vi "Big_LED_control.vi"() -> ()   [LabVIEW 2018]
uses:
  <instrlib>/niDCPower/nidcpower.llb/niDCPower Source Mode.ctl
  <instrlib>/niDCPower/nidcpower.llb/niDCPower Output Function.ctl
  D:/#msp/LV/LED_CONTROL_big_LED_ophir_20.12/AT lib/AmateurStepperMotor.dll
  AT lib/AmateurStepperMotor.dll
  <instrlib>/niDMM/nidmm.llb/niDMM Function.ctl
  <instrlib>/niDMM/nidmm.llb/niDMM Resolution in Digits.ctl
  <vilib>/Instr/_visa.llb/VISA Configure Serial Port (Instr).vi
  <instrlib>/niDMM/nidmm.llb/niDMM Configure Measurement Digits.vi
panel:
  in  "Tab Control 2":enum32{"Шаговик и офир", "Служебная область"}(tab)
  in  "milliseconds to wait":u32=1000
  in  "Go To":dbl
  out "Ophir 1 Char":dbl(graph)=7.0
  in  "DecelerationTime, s":dbl
  in  "AccelerationTime, s":dbl
  in  "HoldOn":bool
  in  "Ophir 1 units":string(combo)="1000" caption="Units"
  out "Ophir 1 Over Range":bool caption="Over Range"
  out "Ophir 1 Optical Power":dbl=7.0 caption="Power" format="%#_4g"
  out "Ophir 1 MAX":dbl=7.0200000000000005 caption="MAX" format="%#_5g"
  in  "Ophir 1 Clear":bool caption="Clear"
  in  "StepMultiplicationFactor":dbl=1.0
  in  "StepDivisor":i32(ring)=8 items=["D1"=1, "D2"=2, "D4"=4, "D8"=8, "D16"=16, "D32"=32]
  in  "Speed":dbl=1000.0
  in  "Погнали!":bool
  in  "Стоп GoTo":bool
  out "Готово":bool
  out "Position":dbl
  in  "Ophir 1 Info":u16(ring)=1 caption="Info" items=["Device : JUNO; s/n:903793", "Head : PD300R-3W   ; s/n:779628"]
  in  "new pos":dbl
  in  "set pos":bool
  out "Device Response":string="*\n"
  in  "Ophir 1 usb channel":i16 caption="usb channel"
  out "Ophir 1 dup Visa Session":refnum<visa-resource-name>="USB0::0x0BD3::0x0777::NI-VISA-60004::RAW" caption="dup Visa Session"
  in  "Ophir 1 Baud Rate (3:9600)":i16(ring)=3 caption="Baud Rate (3:9600)" items=["300", "1200", "4800", "9600", "19200", "38400"]
  out "Ophir 1 Real Optical Power":dbl=0.007 format="%.6e"
  in  "Ophir 1 GPIB Address (10)":string="10" caption="GPIB Address (10)"
  in  "Ophir 1 Port Number (default 2)":i16=1 caption="Port Number (default 2)" min=0 max=20
  in  "Ophir 1 Select Communication Protocol":u16(ring) caption="Select Communication Protocol" items=["USB", "RS232", "GPIB"]
  out "Ophir 1 error out":errorcluster caption="error out"
  in  "Ophir 1 error in (no error)":errorcluster caption="error in (no error)"
  in  "Ophir 1 Wait":u32=100 caption="Wait"
  out "IsOpen":bool=TRUE
  out "Ophir 1 Initialization":bool=TRUE caption="Initialization"
  in  "Tab Control":T1(tab)
  in  "POWER":bool
  in  "Стоп":bool
  in  "Resource Name":refnum<k15>="PXI1Slot2" caption="Источник питания"
  in  "Амперметр":refnum<k15>="PXI1Slot4" caption="NI DMM 1"
  in  "V_MB, V":dbl=5.0 caption="voltage level" format="%_6p"
  in  "curlim_V_MB, A":dbl=0.3 caption="current limit" format="%_6p"
  out "curmes_V_MB, A":dbl caption="measurement" format="%_6g"
  out "chart_0":dbl(graph)=-0.001986406197333734 caption="Waveform Chart 5"
  in  "voltlim_I_LED, V":dbl=2.0 caption="current limit" min=0.01 format="%_6p"
  in  "I_LED, A":dbl=0.005 caption="voltage level" format="%_6p"
  out "chart_1":dbl(graph) caption="Waveform Chart 5"
  out "voltmes_I_LED, V":dbl caption="measurement" format="%_6g"
  out "Current Char":dbl(graph)=0.0019995495676994324
  in  "Arduino":refnum<visa-resource-name>="COM14"
  in  "Сегменты":bool[](array[boolean])=[FALSE, FALSE, FALSE, FALSE, FALSE, FALSE, FALSE, FALSE, FALSE, FALSE, FALSE, FALSE, FALSE, FALSE, FALSE, FALSE, FALSE, FALSE]
  in  "Вольтметр":refnum<k15>="PXI1Slot5" caption="NI DMM 1"
  out "Voltage Char":dbl(graph)=nan
  in  "Port Name":string="COM7" caption="Порт шаговика"
  in  "wave_lenght":string="600"
  in  "Промер":bool caption="Промер сегмента"
  in  "NI DMM 1 Voltage Range 4":string(combo)="-1" caption="Range"
  in  "NI DMM 1 units 4":string(combo)="1" caption="Units"
  out "Voltage":dbl=nan format="%_6g"
  in  "NI DMM 1 Current Range 3":string(combo)="1" caption="Range"
  in  "NI DMM 1 units 3":string(combo)="1000" caption="Units"
  out "Current":dbl=0.0019995495676994324 format="%_6g"
  out "curmes_I_LED, A":dbl caption="measurement" format="%_6g"
  out "voltmes_V_MB, V":dbl caption="measurement" format="%_6g"
  out "Разряд":dbl
  out "+/-":bool
  out "Power off":bool=TRUE
  in  "Command":string="Anode"
  in  "Записать":bool
  out "measure output file refnum":refnum<file>
  out "Voltage, V":dbl=nan caption="Measurement" format="%.5f"
  out "Current, A":dbl=1.9995495676994324e-06 caption="Measurement" format="%.5f"
  out "Тип индикатора":string="Anode"
  out "chart_2":dbl(graph)=4.286668577189643e-07
  in  "V_RES, V":dbl caption="voltage level" format="%_6p"
  out "curmes_V_RES, A":dbl caption="measurement" format="%_6g"
  in  "curlim_V_RES, A":dbl=0.1 caption="current limit" min=0.01 format="%_6p"
  in  "measure path":path=path "D:/NI LabVIEW/MultiOpto/MultiOpto_1.2/Logs/SEL"
  out "Enum":enum16{"Exit", "4", "Промер", "2", "1"}(ring)
  out "№ об-ца":dbl=-1.0
  out "Темп-ра":dbl=-1.0
  out "Сегмент":string
  out "voltmes_V_RES, V":dbl caption="measurement" format="%_6g"
  in  "current level range":dbl format="%#.6p"
  # "Шаговик"
  # "Офир"
  # "Шаговик"
  # "Офир"
  # "position - это значение абсолютное"
  # "j"
  # "c"
  # "d"
  # "e"
  # "g"
  # "h"
  # "a"
  # "b"
  # "f"
  # "k"
  # "L"
  # "m"
  # "n"
  # "p"
  # "dp"
  # "all"
  # "V_MB 5 В\nогрничение 300 м\n\nV_LED 2,1 В\nограничение 200 м"
  # "единицы мА\nrange 1 А"
  # "1. каждый сегмент включаем по отдельности, резистором постраиваем ток до 10 мА\n2. напряжение V_LED при этом не меняется\n3. в такоом положении промеряем сегменты по отдельности\n4. для промера всего индикатора сразу подстраиваем напряжение при неизменном положении резисторов\n5. ток всех индикаторов = ток одного сегмента (10 мА) * число сегментов (15)\n6. добиваемся этого увеличением V_LED"
  # "единицы В\nrange AUTO"
  # "регклировка суммарного тока через индикатор"
  # "24.063\n\n     I          U\n20 мА  1.3 В\n20 мА  1.4 В\n 7 мА   1.15 В"
  # "24.064\n\n     I          U\n10 мА  2 В\n10 мА  2.15 В\n 7 мА   1.9 В"
  # "автоматизировать подбор напряжения по известному максимальному напряжению и току. ОС по току сегмента"
  # "Р1:  +25°C\nР2:  - 60°C\nР3:  +85°C"
  # "регулировать ток в зависимости от температуры.\nс ростом температуры растет ток.\nпид-регулятор??"
  # "0. ввести номер образца\n1. включить нужный сегмент\n2. ввести его в поле справа\n3. вести температуру в поле слева\n4. нажать кнопку \"промер сегмента\""
  # "\"опрашивать кнопки не чаще, чем раз в секунду. сейчас кликать можно чаще, они загорятся, но ничего не произойдет\""
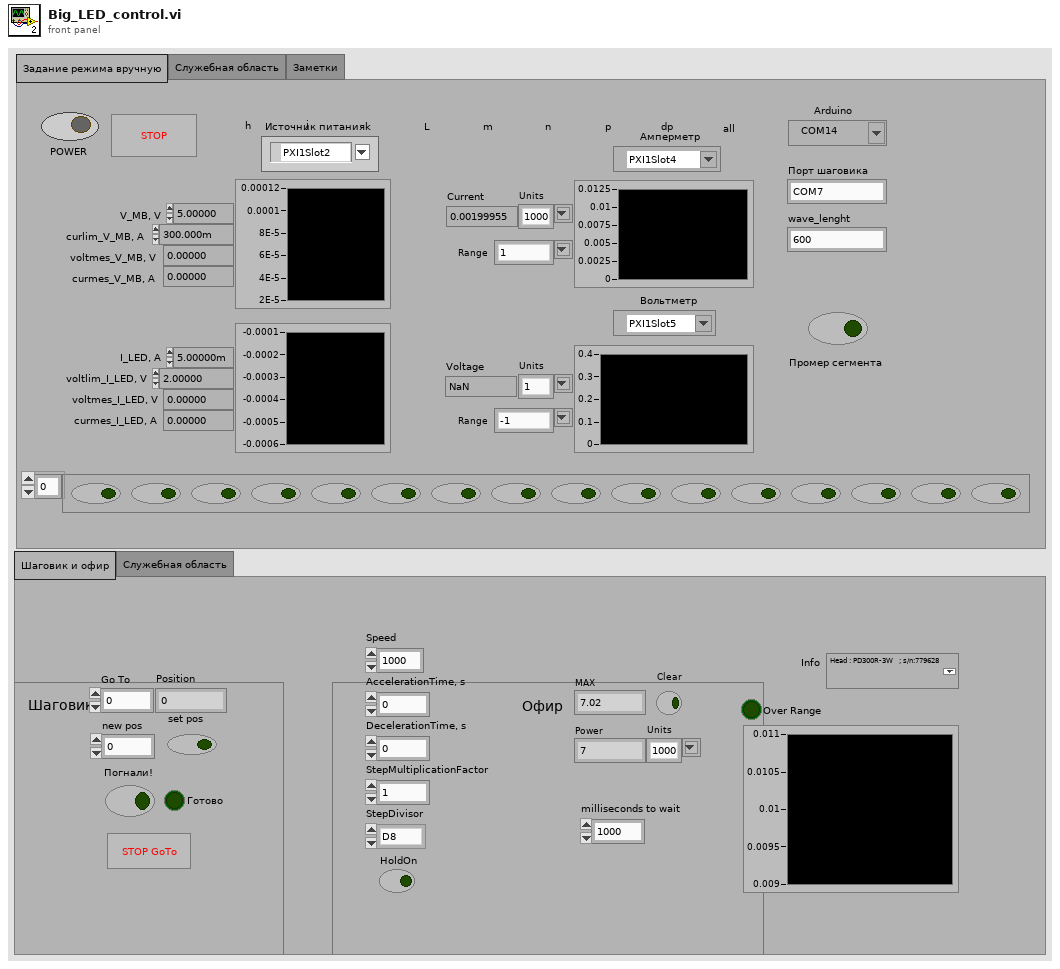
[diagram p1: front panel]
types:
  T1 = enum32{"Задание режима вручную", "Служебная область", "Заметки"}
  T2 = enum16{"open", "replace", "create", "open or create", "replace or create", "replace or create with confirmation"}
  T3 = typedef "niDCPower Output Function.ctl" = i32
  T4 = typedef "niDCPower Source Mode.ctl" = i32
  T5 = typedef "niDMM Function.ctl" = enum16{"DC Volts", "AC Volts", "DC Current", "AC Current", "2-wire Resistance", "4-wire Resistance", "Diode", "Frequency", "Period", "AC Volts DC Coupled", "Capacitance", "Inductance", "Temperature"}
  T6 = typedef "niDMM Resolution in Digits.ctl" = dbl
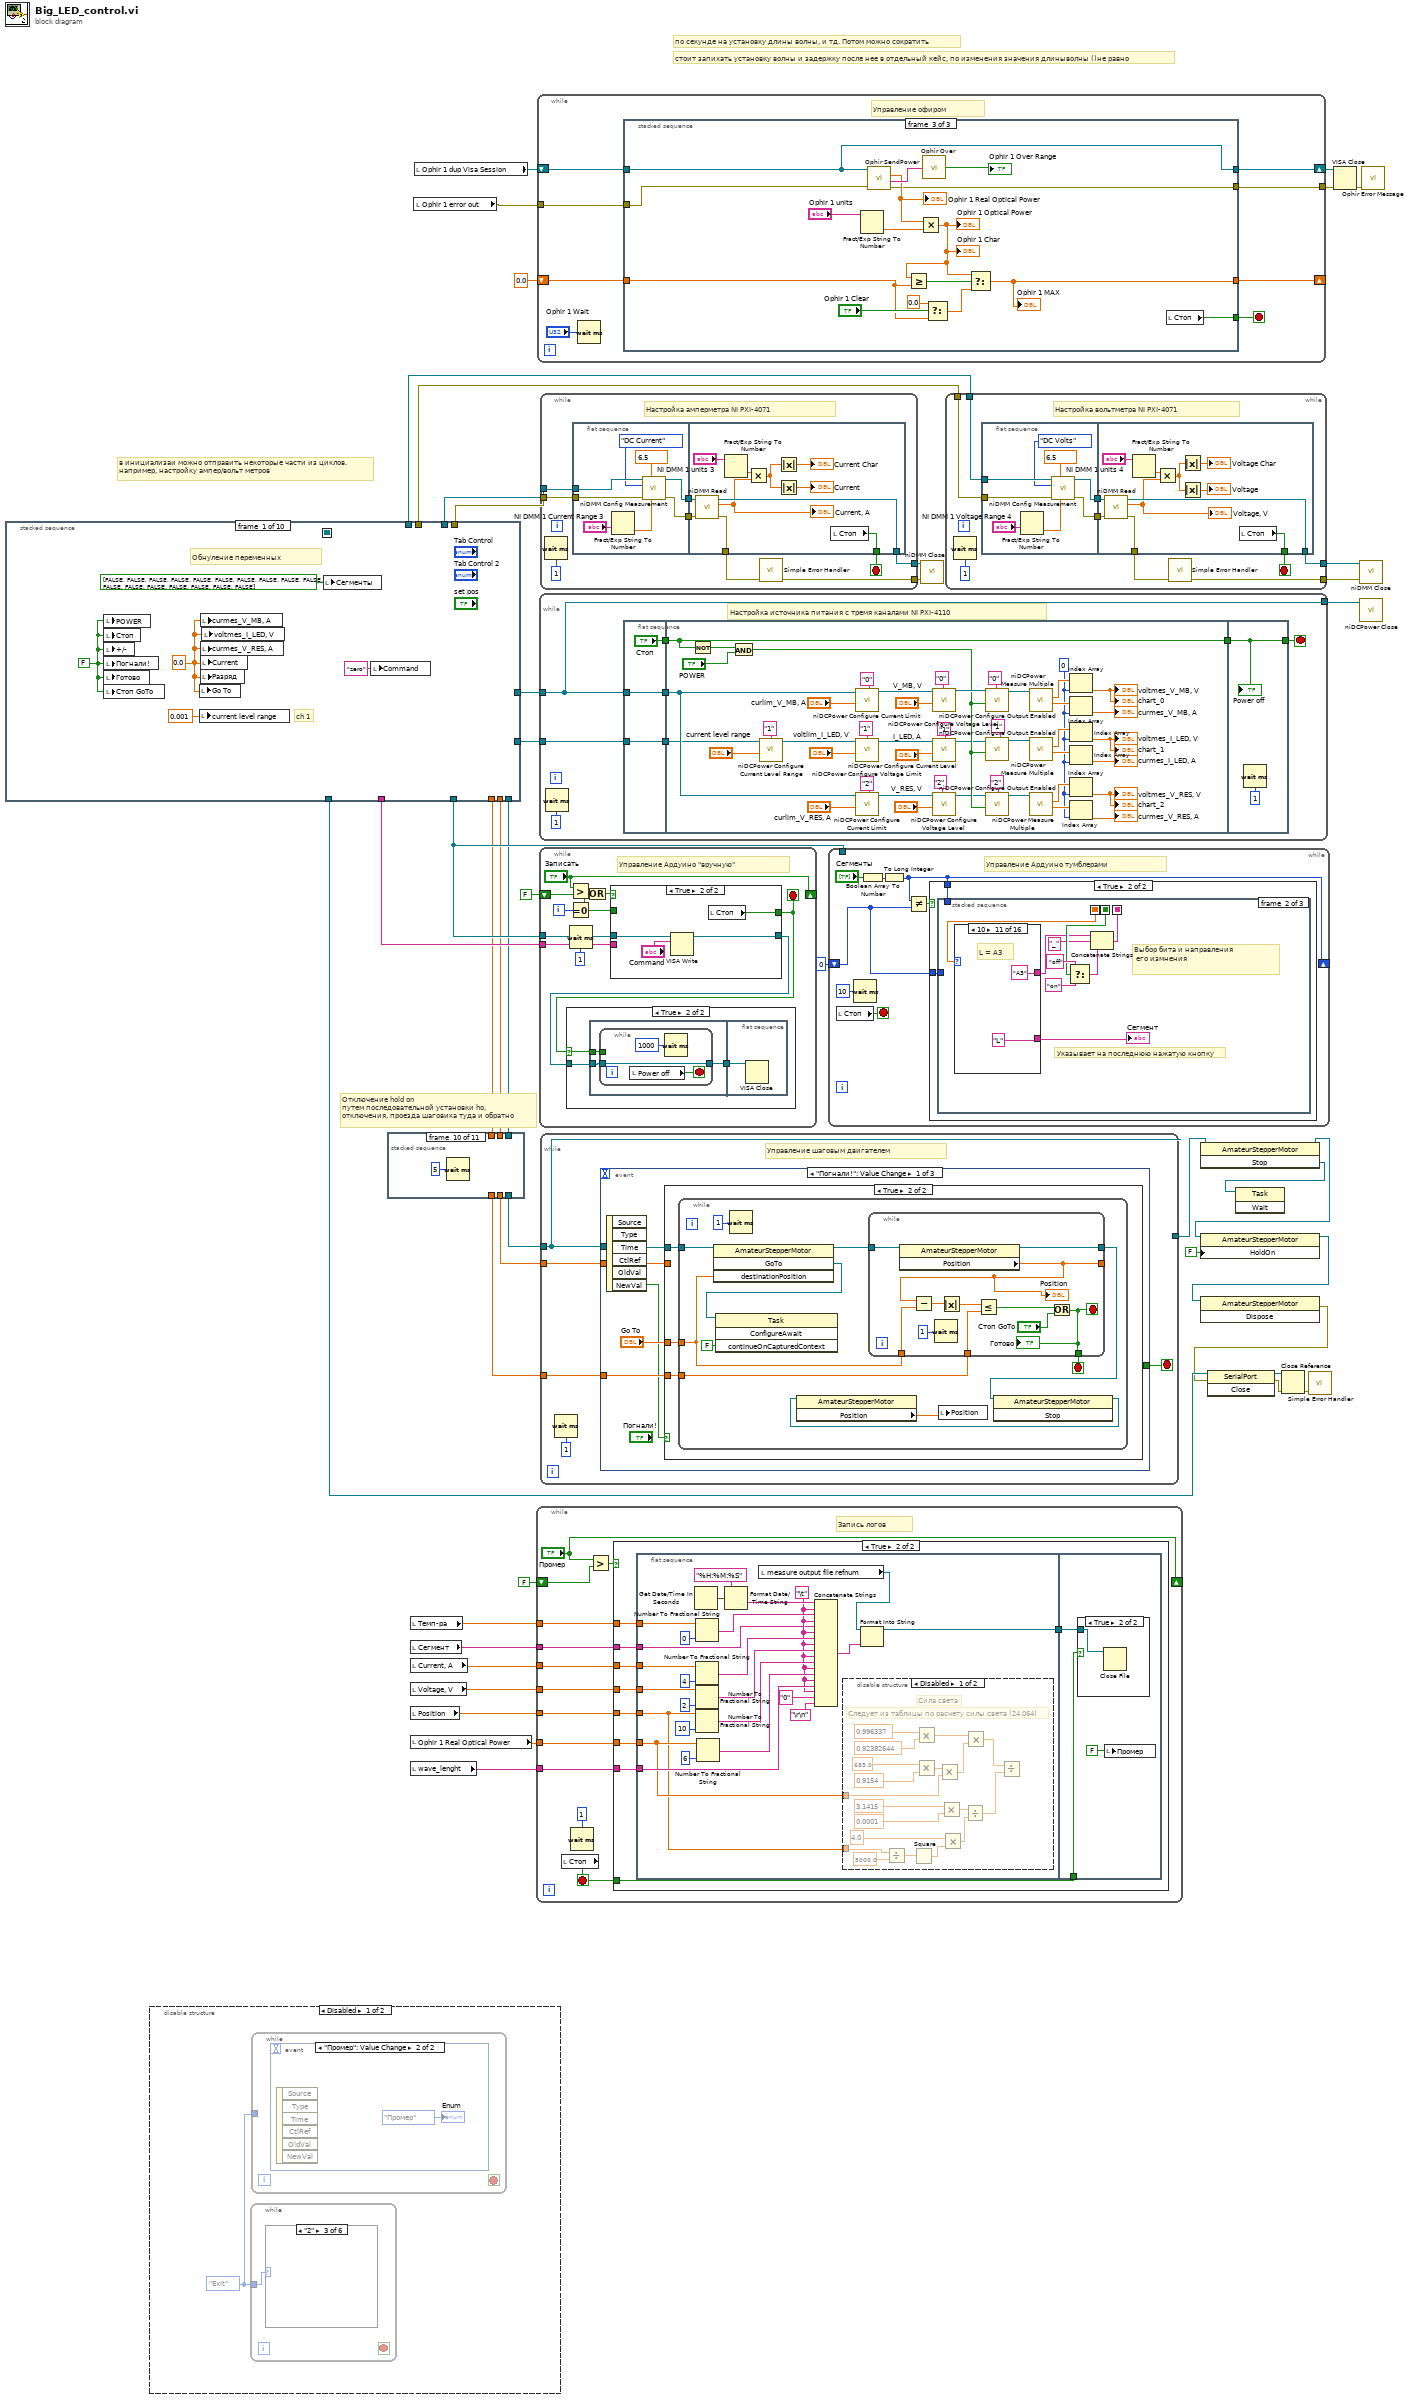
[diagram p0: block diagram]
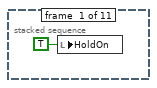
[diagram p2: hidden frame]
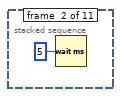
[diagram p3: hidden frame]
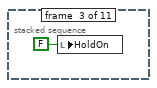
[diagram p4: hidden frame]
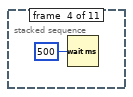
[diagram p5: hidden frame]
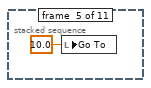
[diagram p6: hidden frame]
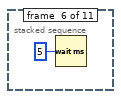
[diagram p7: hidden frame]
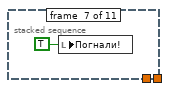
[diagram p8: hidden frame]
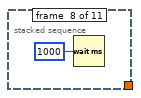
[diagram p9: hidden frame]
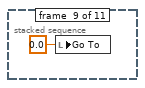
[diagram p10: hidden frame]
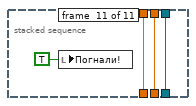
[diagram p11: hidden frame]
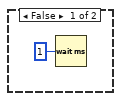
[diagram p12: hidden frame]
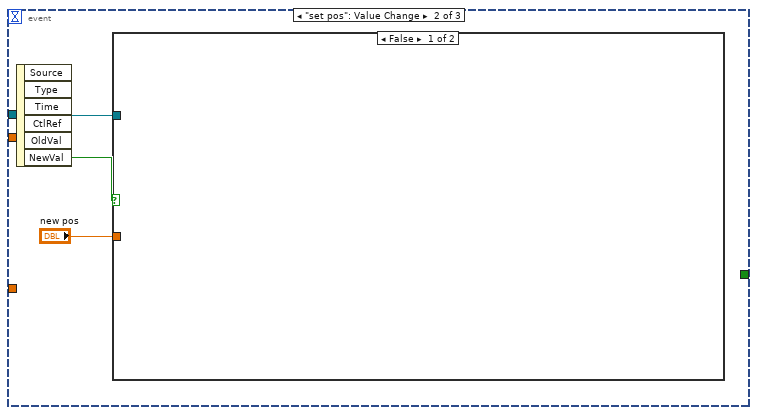
[diagram p13: hidden frame]
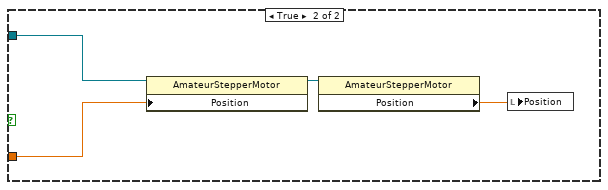
[diagram p14: hidden frame]
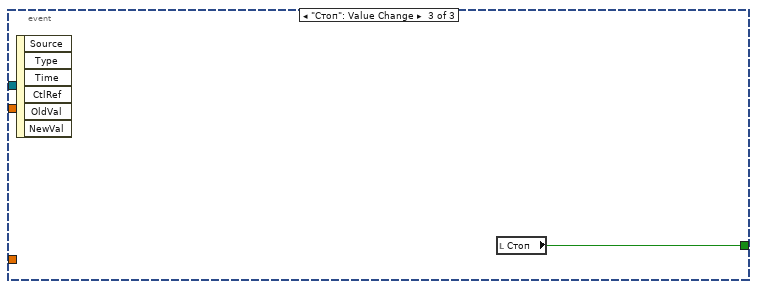
[diagram p15: hidden frame]
diagram:
  # "Отключение hold on\nпутем последовательной установки ho, \nотключения, проезда шаговика туда и обратно"
  # "в инициализаи можно отправить некоторые части из циклов.\nнапример, настройку ампер/вольт метров"
  # "стоит запихать установку волны и задержку после нее в отдельный кейс, по изменения значения длиныволны ()не равно"
  # "по секунде на установку длины волны, и тд. Потом можно сократить"
  n1 = stacked-sequence {
    seq-local: [_ _ _ _ _ _ w104 _ _ _] -> [_ _ _ _ _ _ _ w113 _ _]
    tunnel: [_ _ _ w70 _ _ _ _ _ _] -> w33
    tunnel: [_ w53 _ _ _ _ _ _ _ _] -> w45
    tunnel: [_ w52 _ _ _ _ _ _ _ _] -> w44
    tunnel: [_ _ _ _ w71 _ _ _ _ _] -> w41
    tunnel: [_ _ _ _ _ _ _ _ _ w153] -> w40
    tunnel: [_ _ w56 _ _ _ _ _ _ _] -> w39
    tunnel: [_ _ w55 _ _ _ _ _ _ _] -> w38
    tunnel: [_ _ _ _ _ _ _ w116 _ _] -> w1
    tunnel: [_ _ _ _ _ _ _ w114 _ _] -> w4
    tunnel: [_ _ _ _ _ _ _ w115 _ _] -> w6
    tunnel: [_ _ _ _ _ _ w94 _ _ _] -> w27
    tunnel: [_ _ _ w64 _ _ _ _ _ _] -> w10
    frame #0 {
      w47 = 0.0 ("currentmes_2")
      w48 = FALSE ("Стоп")
      # "ch 1"
      # "Обнуление переменных"
      n2 = local write "POWER"(w48) -> ()
      n3 = local write "Стоп"(w48) -> ()
      n4 = local write "+/-"(w48) -> ()
      n5 = local write "Погнали!"(w48) -> ()
      n6 = local write "Готово"(w48) -> ()
      n7 = local write "Стоп GoTo"(w48) -> ()
      n8 = local write "Go To"(w47) -> ()
      n9 = local write "current level range"(0.001 ("current level range")) -> ()
      n10 = local write "curmes_V_MB, A"(w47) -> ()
      n11 = local write "curmes_V_RES, A"(w47) -> ()
      n12 = local write "Current"(w47) -> ()
      n13 = local write "Разряд"(w47) -> ()
      n14 = local write "voltmes_I_LED, V"(w47) -> ()
      n15 = local write "Сегменты"(bool[] [FALSE, FALSE, FALSE, FALSE, FALSE, FALSE, FALSE, FALSE, FALSE, FALSE, FALSE, FALSE, FALSE, FALSE, FALSE, FALSE, FALSE, FALSE] ("Сегменты")) -> ()
      n16 = local write "Command"("zero" ("Command 2")) -> ()
    }
    frame #1 {
      # "Инициализация амперметра"
      n17 = call <instrlib>:"niDMM Initialize.vi"("Instrument Descriptor"="Амперметр") -> ("error out"=w53:errorcluster, "instrument handle out"=w52:refnum<k15>)  [unwired: 9 in]
    }
    frame #2 {
      # "Инициализация вольтметра"
      n18 = call <instrlib>:"niDMM Initialize.vi"("Instrument Descriptor"="Вольтметр") -> ("error out"=w55:errorcluster, "instrument handle out"=w56:refnum<k15>)  [unwired: 9 in]
    }
    frame #3 {
      w57 = T3 1007 items=["DC Voltage"=1006, "DC Current"=1007, "Pulse Voltage"=1049, "Pulse Current"=1050] ("output function")
      w58 = T3 1006 items=["DC Voltage"=1006, "DC Current"=1007, "Pulse Voltage"=1049, "Pulse Current"=1050] ("output function")
      w62 = T4 1020 items=["Single Point"=1020, "Sequence"=1021] ("source mode")
      # "Инициализация источника питания"
      n19 = call <instrlib>:"niDCPower Initialize.vi"("resource name"="Resource Name") -> ("instrument handle out"=w63:refnum<k15>)  [unwired: 3 in, 7 out]
      n20 = call <instrlib>:"niDCPower Configure Source Mode.vi"("source mode"=w62, "instrument handle"=w63) -> ("instrument handle out"=w61:refnum<k15>)  [unwired: 1 in, 8 out]
      n21 = call <instrlib>:"niDCPower Configure Output Function.vi"("output function"=w57, "instrument handle"=w61) -> ("instrument handle out"=w59:refnum<k15>)  [unwired: 8 in, 1 out]
      n22 = call <instrlib>:"niDCPower Configure Output Function.vi"("output function"=w58, "instrument handle"=w61) -> ("instrument handle out"=w60:refnum<k15>)  [unwired: 8 in, 1 out]
      n23 = call <instrlib>:"niDCPower Configure Voltage Level.vi"("voltage level"=0.0, "channel name"="0,2", "instrument handle"=w60) -> ("instrument handle out"=w70:refnum<k15>)  [unwired: 7 in, 1 out]
      n24 = call <instrlib>:"niDCPower Configure Current Level.vi"("current level"=0.01, "channel name"="1", "instrument handle"=w59) -> ("instrument handle out"=w64:refnum<k15>)  [unwired: 7 in, 1 out]
    }
    frame #4 {
      # "Инициализация Ардуино"
      n25 = call-poly "VISA Configure Serial Port"("VISA resource name"="Arduino", "baud rate (9600)"=u32 9600) -> ("VISA resource name out"=w71:refnum<visa-resource-name>)  [unwired: 12 in, 1 out]
    }
    frame #5 {
      # "Инициализация офира"
      n26 = call "Ophir InitCom.vi"("GPIB Address (default 10)"="Ophir 1 GPIB Address (10)", "Communication (default USB 0)"="Ophir 1 Select Communication Protocol", "USB Channel number (default 0)"="Ophir 1 usb channel", "Port Number (default 2)"="Ophir 1 Port Number (default 2)", "error in (no error)"="Ophir 1 error in (no error)", "Baud Rate (3:9600)"="Ophir 1 Baud Rate (3:9600)") -> ("dup Visa Session"=w80:refnum<visa-resource-name>, "error out"=w79:errorcluster)  [unwired: 1 out]
      n27 = call "Ophir InstrInfo.vi"("Visa Session"=w80, "error in (no error)"=w79) -> ("dup Visa Session"=w92:refnum<visa-resource-name>, "Instrument Info"=w74:string, "error out"=w90:errorcluster)
      n28 = call "Ophir HeadInfo.vi"("Visa Session"=w92, "error in (no error)"=w90) -> ("error out"=w89:errorcluster, "dup Visa Session"=w91:refnum<visa-resource-name>, "Head Info"=w88:string)  [unwired: 6 out]
      n29 = call "Ophir InfoStrings.vi"("error in (no error)"=w89, "Head Info"=w88, "Instrument Info"=w74) -> ("error out"=w87:errorcluster, "Strings Array"=w86:string[])
      n30 = property on="Ophir 1 Info" class="Ring (strict)"("Strings []"=w86) -> ()  [unwired: 2 in, 2 out]
      n31 = call "Ophir ConfigDevice.vi"("Visa Session"=w91, "Measure Choice (0:Power)"=u16 0, "error in (no error)"=w87) -> ("dup Visa Session"=→"Ophir 1 dup Visa Session":refnum<visa-resource-name>, "OK ?"=→"Ophir 1 Initialization":bool, "error out"=→"Ophir 1 error out":errorcluster)  [unwired: 1 out]
    }
    frame #6 {
      w98 = 100 ("WriteTimeout")
      w103 = 1 items=["None", "One", "Two", "OnePointFive"] ("stopBits")
      w100 = 0 items=["None", "Odd", "Even", "Mark", "Space"] ("parity")
      # "убрали открытие порта. шаговик его и так сам откроет"
      # "Инициализация шаговика ч.1"
      n32 = constructor class="SerialPort"("portName"="Port Name", "baudRate"=57600, "parity"=w100, "dataBits"=8, "stopBits"=w103) -> (reference out=w97:refnum<k24>, error out=w96:errorcluster)  [unwired: 3 in, 6 out]
      n33 = property class="SerialPort"(reference=w97, error in=w96, "WriteTimeout"=w98, "ReadTimeout"=w98) -> (reference out=w94:refnum<k24>)  [unwired: 1 out]
      n34 = constructor class="AmateurStepperMotor"("serialPort"=w94) -> (reference out=w104:refnum<k24>, error out=w95:errorcluster)  [unwired: 3 in, 2 out]
      n35 = flat-sequence {
        tunnel: w95 -> [_]
        tunnel: w94 -> [w106]
        frame #0 {
          n36 = property class="SerialPort"(reference=w106) -> ("IsOpen"=→"IsOpen":bool)  [unwired: 1 in, 2 out]
        }
      }
    }
    frame #7 {
      # "стоит допустить изменение\nтих параметров в цикле, а не только \nпри инициализации"
      # "это те самые 50 шагов за мм"
      # "Инициализация шаговика ч.2"
      n37 = property class="AmateurStepperMotor"(reference=w113, "Speed"="Speed", "StepDivisor"="StepDivisor", "StepMultiplicationFactor"="StepMultiplicationFactor", "AccelerationTime"="AccelerationTime, s", "DecelerationTime"="DecelerationTime, s", "HoldOn"="HoldOn") -> (reference out=w116:refnum<k24>, "Position"=w114:dbl, "PositioningPrecision"=w115:dbl)  [unwired: 1 in, 1 out]
    }
    frame #8 {
      w122 = "\t"
      # "Инициализация логов"
      n38 = local read "№ об-ца"() -> (w118:dbl)
      n39 = Number To Fractional String(number=w118, precision (6)=i16 0) -> (F-format string=w119:string)  [unwired: 2 in]
      n40 = Get Date/Time In Seconds() -> (seconds since 1Jan1904=w140:timestamp)
      n41 = Build Path(base path="measure path", name or relative path=w119) -> (appended path=w136:path)
      n42 = call <vilib>:"Check if File or Folder Exists.vi"("path"=w136) -> ("file or folder exists?"=w137:bool, "dup path"=w138:path)  [unwired: 8 in, 1 out]
      n43 = Format Date/Time String(time format string (%c)="MES %d %m %y %H.%M.%S", seconds (now)=w140) -> (date/time string=w141:string)  [unwired: 1 in]
      n44 = case shown="False" w137 {
        tunnel: w138 -> [w149 w150]
        tunnel: [w148 w150] -> w139
        frame False {
          n45 = Create Folder(path (use dialog)=w149) -> (created path=w148:path)  [unwired: 2 in, 2 out]
        }
        frame True {
        }
      }
      n46 = Concatenate Strings(w141, ".xls" ("string")) -> (w142:string)
      n47 = Build Path(base path=w139, name or relative path=w142) -> (appended path=w143:path)
      n48 = Open/Create/Replace File(file path (use dialog)=w143, operation (0:open)=T2."open or create", access (0:read/write)=enum16{"read/write", "read-only", "write-only"}."read/write") -> (refnum out=w144:refnum<file>)  [unwired: 3 in, 2 out]
      n49 = Set File Position(refnum=w144, from (0:start)=enum16{"start", "end", "current"}."end") -> (refnum out=w146:refnum<file>)  [unwired: 2 in, 1 out]
      n50 = Format Into String(initial string=w146, "Time" ("string"), w122, "Temperature, C" ("string"), w122, "Segment" ("string"), w122, "Current, mA" ("string"), w122, "Voltage, V" ("input 7"), w122, "Distance, m" ("string"), w122, "Power, W " ("string"), w122, "Wavelenght, nm" ("input 17"), w122, "Candlepower, kd" ("string"), "\r\n") -> (resulting string=→"measure output file refnum":refnum<file>)  [unwired: 2 in, 1 out]
    }
    frame #9 {
      # "Begin VI: ОК или ОА?"
      n51 = call "Begin.vi"() -> ("Темп-ра"=→"Темп-ра":dbl, "№ об-ца"=→"№ об-ца":dbl, "String"=w153:string)  [unwired: 6 in]
      "Тип индикатора" <- w153
      n52 = local write "Command"(w153) -> ()
    }
  }
  n53 = disable-structure shown="Disabled" {
    frame Disabled {
      w154 = enum16{"Exit", "4", "Промер", "2", "1"}."Exit"
      n54 = while {
        tunnel: w154 -> [w155]
        stop <- _ stop-if-true
        n55 = case shown="\"2\"" w155 {
          frame "Exit", Default {
          }
          frame "4" {
          }
          frame "2" {
          }
          frame "2" {
          }
          frame "1" {
          }
          frame "Промер" {
          }
        }
      }
      n56 = while {
        tunnel: w154 -> [_]
        stop <- _ stop-if-true
        n57 = event shown="[1] \"Промер\": Value Change" {
          selector: _ -> [_ _]
          dyn-events: _ -> [_ _]
          timeout: _ -> [_ _]
          event Timeout {
            n58 = event-data() -> ()  [unwired: 1 in, 3 out]
          }
          event "Промер": Value Change {
            n59 = event-data() -> ()  [unwired: 1 in, 6 out]
            "Enum" <- enum16{"Exit", "4", "Промер", "2", "1"}."Промер" ("Enum")
          }
        }
      }
    }
    frame Enabled {
    }
  }
  n60 = stacked-sequence {
    tunnel: w6 -> [_ _ _ _ _ _ _ _ _ _ w169]
    tunnel: [_ _ _ _ _ _ _ _ _ _ w169] -> w5
    tunnel: w4 -> [_ _ _ _ _ _ _ _ _ _ w168]
    tunnel: [_ _ _ _ _ _ _ _ _ _ w168] -> w3
    tunnel: [_ _ _ _ _ _ _ _ _ _ w167] -> w2
    tunnel: w1 -> [_ _ _ _ _ _ _ _ _ _ w167]
    frame #0 {
      n61 = local write "HoldOn"(TRUE ("HoldOn")) -> ()
    }
    frame #1 {
      n62 = Wait (ms)(milliseconds to wait=u32 5) -> ()  [unwired: 1 out]
    }
    frame #2 {
      n63 = local write "HoldOn"(FALSE ("HoldOn")) -> ()
    }
    frame #3 {
      n64 = Wait (ms)(milliseconds to wait=u32 500) -> ()  [unwired: 1 out]
    }
    frame #4 {
      n65 = local write "Go To"(10.0 ("Go To")) -> ()
    }
    frame #5 {
      n66 = Wait (ms)(milliseconds to wait=u32 5) -> ()  [unwired: 1 out]
    }
    frame #6 {
      n67 = local write "Погнали!"(TRUE ("Погнали!")) -> ()
    }
    frame #7 {
      n68 = Wait (ms)(milliseconds to wait=u32 1000) -> ()  [unwired: 1 out]
    }
    frame #8 {
      n69 = local write "Go To"(0.0 ("Go To")) -> ()
    }
    frame #9 {
      n70 = Wait (ms)(milliseconds to wait=u32 5) -> ()  [unwired: 1 out]
    }
    frame #10 {
      n71 = local write "Погнали!"(TRUE ("Погнали!")) -> ()
    }
  }
  n72 = local read "Темп-ра"() -> (w8:dbl)
  n73 = local read "Сегмент"() -> (w7:string)
  n74 = local read "Current, A"() -> (w26:dbl)
  n75 = local read "Voltage, V"() -> (w25:dbl)
  n76 = local read "Position"() -> (w24:dbl)
  n77 = local read "Ophir 1 Real Optical Power"() -> (w23:dbl)
  n78 = local read "wave_lenght"() -> (w22:string)
  n79 = local read "Ophir 1 error out"() -> (w31:errorcluster)
  n80 = local read "Ophir 1 dup Visa Session"() -> (w32:refnum<visa-resource-name>)
  n81 = while {
    tunnel: w26 -> [w182]
    tunnel: w25 -> [w181]
    tunnel: w24 -> [w180]
    tunnel: w23 -> [w179]
    tunnel: w22 -> [w178]
    shift-right: ["Промер"] -> _
    shift-left: FALSE ("Промер сегмента") -> [w175]
    tunnel: w8 -> [w172]
    tunnel: w7 -> [w171]
    stop <- w173 stop-if-true
    # "Запиcь логов"
    n82 = local read "Стоп"() -> (w173:bool)
    n83 = Wait (ms)(milliseconds to wait=u32 1) -> ()  [unwired: 1 out]
    n84 = Greater?(x="Промер", y=w175) -> (0:w176:bool)
    n85 = case shown="True" w176 {
      tunnel: w182 -> [_ w191]
      tunnel: w181 -> [_ w190]
      tunnel: w180 -> [_ w187]
      tunnel: w179 -> [_ w188]
      tunnel: w178 -> [_ w189]
      tunnel: w173 -> [_ w185]
      tunnel: w172 -> [_ w184]
      tunnel: w171 -> [_ w183]
      frame False {
      }
      frame True {
        n86 = flat-sequence {
          tunnel: w191 -> [w209]
          tunnel: w190 -> [w208]
          tunnel: w189 -> [w206]
          tunnel: w188 -> [w205]
          tunnel: w187 -> [w204]
          tunnel: [w199] -> w186
          tunnel: w184 -> [w198]
          tunnel: w183 -> [w192]
          tunnel: w186 -> [w239]
          tunnel: w185 -> [w238]
          frame #0 {
            w194 = "\t"
            n87 = Get Date/Time In Seconds() -> (seconds since 1Jan1904=w217:timestamp)
            n88 = Number To Fractional String(number=w198, precision (6)=i16 0) -> (F-format string=w196:string)  [unwired: 2 in]
            n89 = Number To Fractional String(number=w209, precision (6)=i16 4) -> (F-format string=w212:string)  [unwired: 2 in]
            n90 = Number To Fractional String(number=w208, precision (6)=i16 2) -> (F-format string=w211:string)  [unwired: 2 in]
            n91 = Number To Fractional String(number=w204, precision (6)=i16 10) -> (F-format string=w210:string)  [unwired: 2 in]
            n92 = Number To Fractional String(number=w205, precision (6)=i16 6) -> (F-format string=w207:string)  [unwired: 2 in]
            n93 = Format Date/Time String(time format string (%c)="%H:%M:%S", seconds (now)=w217) -> (date/time string=w215:string)  [unwired: 1 in]
            n94 = local read "measure output file refnum"() -> (w213:refnum<file>)
            n95 = Concatenate Strings(w215, w194, w196, w194, w192, w194, w212, w194, w211, w194, w210, w194, w207, w194, w206, w194, "0" ("string"), "\r\n") -> (w214:string)
            n96 = disable-structure shown="Disabled" {
              disable-tunnel: w205 -> [w229 _]
              disable-tunnel: w204 -> [w219 _]
              frame Disabled {
                # "Сила света"
                # "Следует из таблицы по расчету силы света (24.064)"
                n97 = Divide(x=w219, y=5000.0) -> (x/y=w221:dbl)
                n98 = Square(x=w221) -> (x^2=w220:dbl)
                n99 = Multiply(x=0.996337, y=0.92382644) -> (x*y=w234:dbl)
                n100 = Multiply(x=683.0, y=0.9154) -> (x*y=w230:dbl)
                n101 = Multiply(x=w230, y=w229) -> (x*y=w228:dbl)
                n102 = Multiply(x=3.1415, y=0.0001) -> (x*y=w224:dbl)
                n103 = Multiply(x=4.0, y=w220) -> (x*y=w223:dbl)
                n104 = Divide(x=w224, y=w223) -> (x/y=w225:dbl)
                n105 = Multiply(x=w234, y=w228) -> (x*y=w233:dbl)
                n106 = Divide(x=w233, y=w225) -> ()  [unwired: 1 out]
              }
              frame Enabled {
              }
            }
            n107 = Format Into String(initial string=w213, w214) -> (resulting string=w199:refnum<file>)  [unwired: 2 in, 1 out]
          }
          frame #1 {
            n108 = case shown="True" w238 {
              tunnel: w239 -> [_ w240]
              frame False {
              }
              frame True {
                n109 = Close File(refnum=w240) -> ()  [unwired: 1 in, 2 out]
              }
            }
            n110 = local write "Промер"(FALSE ("Промер")) -> ()
          }
        }
      }
    }
  }
  n111 = while {
    tunnel: w31 -> [w247]
    shift-right: [w243] -> _
    shift-left: 0.0 ("t") -> [w246]
    shift-right: [w244] -> w20
    shift-left: w32 -> [w248]
    tunnel: [w242] -> w19
    stop <- w241 stop-if-true
    # "Управление офиром"
    n112 = Wait (ms)(milliseconds to wait="Ophir 1 Wait") -> ()  [unwired: 1 out]
    n113 = stacked-sequence {
      tunnel: w248 -> [w252 _ w255]
      tunnel: w247 -> [w251 _ w257]
      tunnel: w246 -> [_ _ w258]
      tunnel: [_ _ w255] -> w244
      tunnel: [_ _ w259] -> w243
      tunnel: [_ _ w256] -> w242
      tunnel: [_ _ w254] -> w241
      frame #0 {
        n114 = call "light_setWaveLenght.vi"("error in (no error)"=w251, "Visa Session"=w252, "wave_lenght"="wave_lenght") -> ("Device Response"=→"Device Response":string)  [unwired: 6 in, 2 out]
      }
      frame #1 {
        n115 = Wait (ms)(milliseconds to wait="milliseconds to wait") -> ()  [unwired: 1 out]
      }
      frame #2 {
        n116 = Fract/Exp String To Number(string="Ophir 1 units") -> (number=w262:dbl)  [unwired: 3 in, 1 out]
        n117 = call "Ophir SendPower.vi"("Visa Session"=w255, "error in (no error)"=w257) -> ("Value Number"=w261:dbl, "Value String"=w268:string, "error out"=w256:errorcluster)  [unwired: 1 out]
        "Ophir 1 Real Optical Power" <- w261
        n118 = Multiply(x=w261, y=w262) -> (x*y=w265:dbl)
        "Ophir 1 Char" <- w265
        "Ophir 1 Optical Power" <- w265
        n119 = Greater Or Equal?(x=w265, y=w258) -> (x >= y?=w266:bool)
        n120 = call "Ophir Over.vi"("Value String"=w268) -> ("Overrange"=→"Ophir 1 Over Range":bool)
        n121 = Select(t=0.0, s="Ophir 1 Clear", f=w258) -> (s? t:f=w264:dbl)
        n122 = Select(t=w265, s=w266, f=w264) -> (s? t:f=w259:dbl)
        "Ophir 1 MAX" <- w259
        n123 = local read "Стоп"() -> (w254:bool)
      }
    }
  }
  n124 = while {
    tunnel: w33 -> [w274]
    tunnel: [w274] -> w42
    tunnel: w10 -> [w271]
    stop <- w270 stop-if-true
    # "Настройка источника питания с тремя каналами NI PXI-4110"
    n125 = Wait (ms)(milliseconds to wait=u32 1) -> ()  [unwired: 1 out]
    n126 = flat-sequence {
      tunnel: w274 -> [w280]
      tunnel: [w280] -> w276
      tunnel: ["Стоп"] -> w275
      tunnel: [w278] -> w272
      tunnel: w271 -> [w278]
      tunnel: w276 -> [w322]
      tunnel: w275 -> [w326]
      tunnel: [w326] -> w273
      tunnel: w272 -> [w284]
      tunnel: [w328] -> w270
      tunnel: w273 -> [w328]
      frame #0 {
      }
      frame #1 {
        w291 = 0 ("index")
        n127 = Not(x=w326) -> (.not. x?=w325:bool)
        n128 = And(x=w325, y="POWER") -> (x .and. y?=w321:bool)
        n129 = call <instrlib>:"niDCPower Configure Current Level Range.vi"("current level range"="current level range", "channel name"="1", "instrument handle"=w284) -> ("instrument handle out"=w283:refnum<k15>)  [unwired: 7 in, 1 out]
        n130 = call <instrlib>:"niDCPower Configure Current Limit.vi"("current limit"="curlim_V_MB, A", "channel name"="0", "instrument handle"=w322) -> ("instrument handle out"=w312:refnum<k15>)  [unwired: 7 in, 1 out]
        n131 = call <instrlib>:"niDCPower Configure Voltage Limit.vi"("voltage limit"="voltlim_I_LED, V", "channel name"="1", "instrument handle"=w283) -> ("instrument handle out"=w316:refnum<k15>)  [unwired: 7 in, 1 out]
        n132 = call <instrlib>:"niDCPower Configure Current Limit.vi"("current limit"="curlim_V_RES, A", "channel name"="2", "instrument handle"=w322) -> ("instrument handle out"=w306:refnum<k15>)  [unwired: 7 in, 1 out]
        n133 = call <instrlib>:"niDCPower Configure Voltage Level.vi"("voltage level"="V_MB, V", "channel name"="0", "instrument handle"=w312) -> ("instrument handle out"=w323:refnum<k15>)  [unwired: 7 in, 1 out]
        n134 = call <instrlib>:"niDCPower Configure Current Level.vi"("current level"="I_LED, A", "channel name"="1", "instrument handle"=w316) -> ("instrument handle out"=w317:refnum<k15>)  [unwired: 7 in, 1 out]
        n135 = call <instrlib>:"niDCPower Configure Voltage Level.vi"("voltage level"="V_RES, V", "channel name"="2", "instrument handle"=w306) -> ("instrument handle out"=w307:refnum<k15>)  [unwired: 7 in, 1 out]
        n136 = call <instrlib>:"niDCPower Configure Output Enabled.vi"("output enabled"=w321, "channel name"="0", "instrument handle"=w323) -> ("instrument handle out"=w300:refnum<k15>)  [unwired: 7 in, 1 out]
        n137 = call <instrlib>:"niDCPower Configure Output Enabled.vi"("output enabled"=w321, "channel name"="1", "instrument handle"=w317) -> ("instrument handle out"=w293:refnum<k15>)  [unwired: 7 in, 1 out]
        n138 = call <instrlib>:"niDCPower Configure Output Enabled.vi"("output enabled"=w321, "channel name"="2", "instrument handle"=w307) -> ("instrument handle out"=w292:refnum<k15>)  [unwired: 7 in, 1 out]
        n139 = call <instrlib>:"niDCPower Measure Multiple.vi"("instrument handle"=w300) -> ("current measurements"=w298:dbl[], "voltage measurements"=w299:dbl[])  [unwired: 7 in, 2 out]
        n140 = call <instrlib>:"niDCPower Measure Multiple.vi"("instrument handle"=w293) -> ("current measurements"=w296:dbl[], "voltage measurements"=w297:dbl[])  [unwired: 7 in, 2 out]
        n141 = call <instrlib>:"niDCPower Measure Multiple.vi"("instrument handle"=w292) -> ("current measurements"=w294:dbl[], "voltage measurements"=w295:dbl[])  [unwired: 7 in, 2 out]
        n142 = Index Array(array=w299, index=w291) -> (element=→"chart_0" →"voltmes_V_MB, V":dbl)
        n143 = Index Array(array=w298, index=w291) -> (element=→"curmes_V_MB, A":dbl)
        n144 = Index Array(array=w297, index=w291) -> (element=→"chart_1" →"voltmes_I_LED, V":dbl)
        n145 = Index Array(array=w296, index=w291) -> (element=→"curmes_I_LED, A":dbl)
        n146 = Index Array(array=w295, index=w291) -> (element=→"chart_2" →"voltmes_V_RES, V":dbl)
        n147 = Index Array(array=w294, index=w291) -> (element=→"curmes_V_RES, A":dbl)
      }
      frame #2 {
        n148 = Wait (ms)(milliseconds to wait=u32 1) -> ()  [unwired: 1 out]
        "Power off" <- w328
      }
    }
  }
  n149 = while {
    tunnel: w41 -> [w336]
    shift-right: ["Записать"] -> _
    shift-left: FALSE ("Записать") -> [w338]
    tunnel: w40 -> [w334]
    i -> [w335]
    stop <- w329 stop-if-true
    # "Управление Ардуино \"вручную\""
    n150 = Greater?(x="Записать", y=w338) -> (0:w332:bool)
    n151 = Equal To 0?(x=w335) -> (x = 0?=w331:bool)
    n152 = Wait (ms)(milliseconds to wait=u32 1) -> ()  [unwired: 1 out]
    n153 = Or(x=w332, y=w331) -> (x .or. y?=w333:bool)
    n154 = case shown="True" w333 {
      tunnel: w336 -> [w350 w355]
      tunnel: [w351 w354] -> w329
      tunnel: w334 -> [_ _]
      tunnel: w331 -> [_ _]
      tunnel: [w350 w352] -> w330
      frame False {
        n155 = local read "Стоп"() -> (w351:bool)
      }
      frame True {
        n156 = VISA Write(VISA resource name=w355, write buffer="Command") -> (VISA resource name out=w352:refnum<visa-resource-name>)  [unwired: 1 in, 2 out]
        n157 = local read "Стоп"() -> (w354:bool)
      }
    }
    n158 = case shown="True" w329 {
      selector: w329 -> [_ w340]
      tunnel: w330 -> [_ w342]
      frame False {
      }
      frame True {
        n159 = flat-sequence {
          tunnel: w342 -> [w345]
          tunnel: [w344] -> w341
          tunnel: w340 -> [w343]
          tunnel: w341 -> [w349]
          frame #0 {
            n160 = while {
              tunnel: w345 -> [w348]
              tunnel: [w348] -> w344
              tunnel: w343 -> [_]
              stop <- w346 stop-if-true
              n161 = local read "Power off"() -> (w346:bool)
              n162 = Wait (ms)(milliseconds to wait=u32 1000) -> ()  [unwired: 1 out]
            }
          }
          frame #1 {
            n163 = VISA Close(VISA resource name=w349) -> ()  [unwired: 1 in, 1 out]
          }
        }
      }
    }
  }
  n164 = while {
    tunnel: [w362] -> w34
    tunnel: w44 -> [w360]
    tunnel: w45 -> [w359]
    tunnel: [w356] -> w35
    stop <- w358 stop-if-true
    # "Настройка амперметра NI PXI-4071"
    n165 = Wait (ms)(milliseconds to wait=u32 1) -> ()  [unwired: 1 out]
    n166 = flat-sequence {
      tunnel: [w369] -> w364
      tunnel: w360 -> [w367]
      tunnel: w359 -> [w371]
      tunnel: [w368] -> w363
      tunnel: w364 -> [w380]
      tunnel: w363 -> [w383]
      tunnel: [w379] -> w358
      tunnel: [w378] -> w356
      tunnel: [w377] -> w357
      frame #0 {
        w365 = T6 6.5 items=["3 1/2"=3.5, "4 1/2"=4.5, "5 1/2"=5.5, "6 1/2"=6.5, "7 1/2"=7.5] ("Resolution in Digits")
        n167 = Fract/Exp String To Number(string="NI DMM 1 Current Range 3") -> (number=w370:dbl)  [unwired: 3 in, 1 out]
        n168 = call-poly <instrlib>:"niDMM Config Measurement.vi"("Range"=w370, "Resolution in Digits"=w365, "error in (no error)"=w371, "Function"=niDMM_Function."DC Current" ("Measurement Type"), "instrument handle"=w367) -> ("error out"=w368:errorcluster, "instrument handle out"=w369:refnum<k15>)  [unwired: 5 in]
      }
      frame #1 {
        n169 = call <instrlib>:"niDMM Read.vi"("error in (no error)"=w383, "instrument handle"=w380) -> ("error out"=w377:errorcluster, "Measurement"=w373:dbl, "instrument handle out"=w378:refnum<k15>)  [unwired: 7 in]
        "Current, A" <- w373
        n170 = Fract/Exp String To Number(string="NI DMM 1 units 3") -> (number=w381:dbl)  [unwired: 3 in, 1 out]
        n171 = Multiply(x=w381, y=w373) -> (x*y=w374:dbl)
        n172 = Absolute Value(x=w374) -> (abs(x)=→"Current Char":dbl)
        n173 = Absolute Value(x=w374) -> (abs(x)=→"Current":dbl)
        n174 = local read "Стоп"() -> (w379:bool)
      }
    }
    n175 = call <vilib>:"Simple Error Handler.vi"("error in (no error)"=w357) -> ("error out"=w362:errorcluster)  [unwired: 1 in, 7 out]
  }
  n176 = while {
    tunnel: w2 -> [w385]
    tunnel: w5 -> [w387]
    tunnel: [w385] -> w9
    tunnel: w3 -> [w388]
    stop <- w384 stop-if-true
    # "Управление шаговым двигателем"
    n177 = Wait (ms)(milliseconds to wait=u32 1) -> ()  [unwired: 1 out]
    n178 = event shown="[0] \"Погнали!\": Value Change" {
      selector: _ -> [_ _ _]
      dyn-events: _ -> [_ _ _]
      timeout: _ -> [_ _ _]
      tunnel: w385 -> [w393 w421 _]
      tunnel: w388 -> [w392 _ _]
      tunnel: w387 -> [w391 _ _]
      tunnel: [_ _ w427] -> w384
      event "Погнали!": Value Change {
        n179 = event-data() -> ("NewVal"=w389:bool)  [unwired: 1 in, 5 out]
        n180 = case shown="True" w389 {
          tunnel: "Go To" -> [_ w397]
          tunnel: w393 -> [_ w396]
          tunnel: w392 -> [_ _]
          tunnel: w391 -> [_ w395]
          frame False {
            n181 = Wait (ms)(milliseconds to wait=u32 1) -> ()  [unwired: 1 out]
          }
          frame True {
            n182 = while {
              tunnel: w397 -> [w404]
              tunnel: w396 -> [w405]
              tunnel: w395 -> [w407]
              stop <- w408 stop-if-true
              n183 = invoke class="AmateurStepperMotor" method="GoTo"(reference=w405, "destinationPosition"=w404) -> (reference out=w400:refnum<k24>, "GoTo"=w403:refnum<k24>)  [unwired: 2 in, 2 out]
              n184 = invoke class="Task" method="ConfigureAwait"(reference=w403, "continueOnCapturedContext"=FALSE) -> ()  [unwired: 2 in, 4 out]
              n185 = Wait (ms)(milliseconds to wait=u32 1) -> ()  [unwired: 1 out]
              n186 = while {
                tunnel: [w409] -> _
                tunnel: [w411] -> w401
                tunnel: [w413] -> w408
                tunnel: w404 -> [w418]
                tunnel: w407 -> [w416]
                tunnel: w400 -> [w410]
                stop <- w413 stop-if-true
                n187 = property class="AmateurStepperMotor"(reference=w410) -> (reference out=w411:refnum<k24>, "Position"=w409:dbl)  [unwired: 1 in, 1 out]
                "Position" <- w409
                n188 = Subtract(x=w409, y=w418) -> (x-y=w419:dbl)
                n189 = Wait (ms)(milliseconds to wait=u32 1) -> ()  [unwired: 1 out]
                n190 = Absolute Value(x=w419) -> (abs(x)=w417:dbl)
                n191 = Less Or Equal?(x=w417, y=w416) -> (x <= y?=w415:bool)
                n192 = Or(x=w415, y="Стоп GoTo") -> (x .or. y?=w413:bool)
                "Готово" <- w413
              }
              n193 = invoke class="AmateurStepperMotor" method="Stop"(reference=w401) -> (reference out=w399:refnum<k24>)  [unwired: 2 in, 2 out]
              n194 = property class="AmateurStepperMotor"(reference=w399) -> ("Position"=w398:dbl)  [unwired: 1 in, 2 out]
              n195 = local write "Position"(w398) -> ()
            }
          }
        }
      }
      event "set pos": Value Change {
        n196 = event-data() -> ("NewVal"=w422:bool)  [unwired: 1 in, 5 out]
        n197 = case shown="False" w422 {
          tunnel: w421 -> [_ w426]
          tunnel: "new pos" -> [_ w425]
          frame False {
          }
          frame True {
            n198 = property class="AmateurStepperMotor"(reference=w426, "Position"=w425) -> (reference out=w424:refnum<k24>)  [unwired: 1 in, 1 out]
            n199 = property class="AmateurStepperMotor"(reference=w424) -> ("Position"=w423:dbl)  [unwired: 1 in, 2 out]
            n200 = local write "Position"(w423) -> ()
          }
        }
      }
      event "Стоп": Value Change {
        n201 = event-data() -> ()  [unwired: 1 in, 6 out]
        n202 = local read "Стоп"() -> (w427:bool)
      }
    }
  }
  n203 = while {
    shift-right: [w430] -> _
    shift-left: 0 -> [w431]
    tunnel: w41 -> [_]
    stop <- w434 stop-if-true
    # "Управление Ардуино тумблерами"
    n204 = local read "Стоп"() -> (w434:bool)
    n205 = Wait (ms)(milliseconds to wait=u32 10 ("millisecond timer value")) -> ()  [unwired: 1 out]
    n206 = Boolean Array To Number(Boolean array="Сегменты") -> (number=w429:u32)
    n207 = To Long Integer(number=w429) -> (32bit integer=w430:i32)
    n208 = Not Equal?(x=w430, y=w431) -> (x != y?=w432:bool)
    n209 = case shown="True" w432 {
      tunnel: w430 -> [_ w435]
      tunnel: w431 -> [_ w436]
      frame False {
      }
      frame True {
        n210 = stacked-sequence {
          seq-local: [w439 _ _] -> [_ w450 _]
          seq-local: [w437 _ _] -> [_ w445 _]
          seq-local: [_ w446 _] -> [_ _ w486]
          tunnel: w435 -> [w441 _ _]
          tunnel: w436 -> [w440 _ _]
          frame #0 {
            # "Детектирвоание позиции и\nнаправления изменения бита"
            n211 = Subtract(x=w441, y=w440) -> (x-y=w442:i32)
            n212 = To Double Precision Float(number=w442) -> (double precision float=w443:dbl)
            n213 = Greater Than 0?(x=w442) -> (x > 0?=w439:bool)
            "+/-" <- w439
            n214 = Absolute Value(x=w443) -> (abs(x)=w438:dbl)
            n215 = Logarithm Base 2(1:w438) -> (0:w437:dbl)
            "Разряд" <- w437
          }
          frame #1 {
            # "Указывает на последнюю нажатую кнопку"
            # "Выбор бита и направления\n его измнения"
            n216 = case shown="10" w445 {
              tunnel: ["D10" "D9" "D5" "D8" "D11" "D12" "A1" "D4" "A5" "A4" "A3" "A2" "A0" "D13" "D3" "All"] -> w448
              tunnel: ["a" "b" "c" "d" "e" "f" "g" "h" "j" "k" "L" "m" "n" "p" "dp" "All"] -> w444
              frame 0, Default {
                # "a = D10"
              }
              frame 1 {
                # "b = D9"
              }
              frame 2 {
                # "c = D5"
              }
              frame 3 {
                # "d = D8"
              }
              frame 4 {
                # "e = D11"
              }
              frame 5 {
                # "f = D12"
              }
              frame 6 {
                # "g = A1"
              }
              frame 7 {
                # "h = D4"
              }
              frame 8 {
                # "j = A5"
              }
              frame 9 {
                # "k = A4"
              }
              frame 10 {
                # "L = A3"
              }
              frame 11 {
                # "m = A2"
              }
              frame 12 {
                # "n = A0"
              }
              frame 13 {
                # "p = D13"
              }
              frame 14 {
                # "dp = D3"
              }
              frame 15 {
              }
            }
            "Сегмент" <- w444
            n217 = Select(t="off", s=w450, f="on") -> (s? t:f=w447:string)
            n218 = Concatenate Strings(w448, "_" ("string"), w447) -> (w446:string)
          }
          frame #2 {
            # "Передача команды в Ардуино"
            n219 = Equal?(x=w486, y="All_off") -> (x = y?=w489:bool)
            n220 = Equal?(x=w486, y="All_on") -> (x = y?=w487:bool)
            n221 = case shown="True" w489 {
              frame False {
              }
              frame True {
                n222 = local write "Сегменты"(bool[] [TRUE, TRUE, TRUE, TRUE, TRUE, TRUE, TRUE, TRUE, TRUE, TRUE, TRUE, TRUE, TRUE, TRUE, TRUE, TRUE] ("Сегменты")) -> ()
              }
            }
            n223 = case shown="True" w487 {
              frame False {
              }
              frame True {
                n224 = local write "Сегменты"(bool[] [FALSE, FALSE, FALSE, FALSE, FALSE, FALSE, FALSE, FALSE, FALSE, FALSE, FALSE, FALSE, FALSE, FALSE, FALSE, FALSE] ("Сегменты")) -> ()
              }
            }
            n225 = stacked-sequence {
              tunnel: w486 -> [w492 _ _]
              frame #0 {
                n226 = local write "Command"(w492) -> ()
              }
              frame #1 {
                n227 = local write "Записать"(TRUE ("Записать")) -> ()
                n228 = Wait (ms)(milliseconds to wait=u32 1000) -> ()  [unwired: 1 out]
              }
              frame #2 {
                n229 = local write "Записать"(FALSE ("Записать")) -> ()
                n230 = Wait (ms)(milliseconds to wait=u32 1000) -> ()  [unwired: 1 out]
              }
            }
          }
        }
      }
    }
  }
  n231 = call <instrlib>:"niDMM Close.vi"("error in (no error)"=w34, "instrument handle"=w35) -> ()  [unwired: 9 in, 1 out]
  n232 = while {
    tunnel: [w503] -> w36
    tunnel: w39 -> [w501]
    tunnel: w38 -> [w500]
    tunnel: [w497] -> w37
    stop <- w499 stop-if-true
    # "Настройка вольтметра NI PXI-4071"
    n233 = Wait (ms)(milliseconds to wait=u32 1) -> ()  [unwired: 1 out]
    n234 = flat-sequence {
      tunnel: [w510] -> w505
      tunnel: w501 -> [w508]
      tunnel: w500 -> [w512]
      tunnel: [w509] -> w504
      tunnel: w505 -> [w521]
      tunnel: w504 -> [w524]
      tunnel: [w520] -> w499
      tunnel: [w519] -> w497
      tunnel: [w518] -> w498
      frame #0 {
        w506 = T6 6.5 items=["3 1/2"=3.5, "4 1/2"=4.5, "5 1/2"=5.5, "6 1/2"=6.5, "7 1/2"=7.5] ("Resolution in Digits")
        n235 = Fract/Exp String To Number(string="NI DMM 1 Voltage Range 4") -> (number=w511:dbl)  [unwired: 3 in, 1 out]
        n236 = call-poly <instrlib>:"niDMM Config Measurement.vi"("Range"=w511, "Resolution in Digits"=w506, "error in (no error)"=w512, "Function"=niDMM_Function."DC Volts" ("Measurement Type"), "instrument handle"=w508) -> ("error out"=w509:errorcluster, "instrument handle out"=w510:refnum<k15>)  [unwired: 5 in]
      }
      frame #1 {
        n237 = call <instrlib>:"niDMM Read.vi"("error in (no error)"=w524, "instrument handle"=w521) -> ("error out"=w518:errorcluster, "Measurement"=w516:dbl, "instrument handle out"=w519:refnum<k15>)  [unwired: 7 in]
        "Voltage, V" <- w516
        n238 = Fract/Exp String To Number(string="NI DMM 1 units 4") -> (number=w522:dbl)  [unwired: 3 in, 1 out]
        n239 = Multiply(x=w522, y=w516) -> (x*y=w514:dbl)
        n240 = Absolute Value(x=w514) -> (abs(x)=→"Voltage Char":dbl)
        n241 = Absolute Value(x=w514) -> (abs(x)=→"Voltage":dbl)
        n242 = local read "Стоп"() -> (w520:bool)
      }
    }
    n243 = call <vilib>:"Simple Error Handler.vi"("error in (no error)"=w498) -> ("error out"=w503:errorcluster)  [unwired: 1 in, 7 out]
  }
  n244 = invoke class="AmateurStepperMotor" method="Stop"(reference=w9) -> (reference out=w16:refnum<k24>, "Stop"=w17:refnum<k24>)  [unwired: 2 in, 1 out]
  n245 = property class="AmateurStepperMotor"(reference=w16, "HoldOn"=FALSE) -> (reference out=w15:refnum<k24>)  [unwired: 1 in, 1 out]
  n246 = invoke class="AmateurStepperMotor" method="Dispose"(reference=w15) -> (error out=w12:errorcluster)  [unwired: 2 in, 2 out]
  n247 = invoke class="SerialPort" method="Close"(reference=w27, error in=w12) -> (reference out=w11:refnum<k24>, error out=w13:errorcluster)  [unwired: 1 in, 1 out]
  n248 = invoke class="Task" method="Wait"(reference=w17) -> ()  [unwired: 2 in, 3 out]
  n249 = Close Reference(reference=w11, error in (no error)=w13) -> (error out=w14:errorcluster)
  n250 = call <vilib>:"Simple Error Handler.vi"("error in (no error)"=w14) -> ()  [unwired: 1 in, 8 out]
  n251 = VISA Close(VISA resource name=w20, error in (no error)=w19) -> (error out=w29:errorcluster)
  n252 = call <instrlib>:"niDMM Close.vi"("error in (no error)"=w36, "instrument handle"=w37) -> ()  [unwired: 9 in, 1 out]
  n253 = call <instrlib>:"niDCPower Close.vi"("instrument handle"=w42) -> ()  [unwired: 10 in, 1 out]
  n254 = call "Ophir Error Message.vi"("error in (no error)"=w29) -> ()  [unwired: 3 in, 4 out]
